vi "Error Query.vi"(8 "error in (no error)":errorcluster, 11 "VISA resource name":refnum<visa-resource-name>) -> (0 "error out":errorcluster, 1 "Error Message":string, 2 "Error Code":i32[](array[numeric]), 3 "VISA resource name out":refnum<visa-resource-name>)   [LabVIEW 2015, in "ZhiYuan ZDS Series for TCP.lvlib"]
doc: "Queries the instrument for any errors in the instrument's error queue. It will continue to read errors until all errors have been read from the instrument. Any errors will be returned in the <B>error out</B> control.\n\n<B>Note:</B>\nThis VI is called automatically by most driver VIs so it is not usually necessary to call this in an application."
uses:
  ZhiYuan ZDS Series for TCP.lvlib
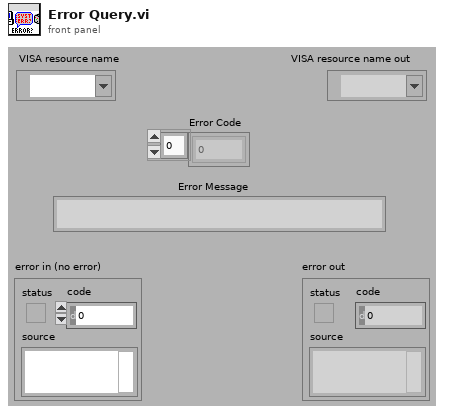
[diagram p1: front panel]
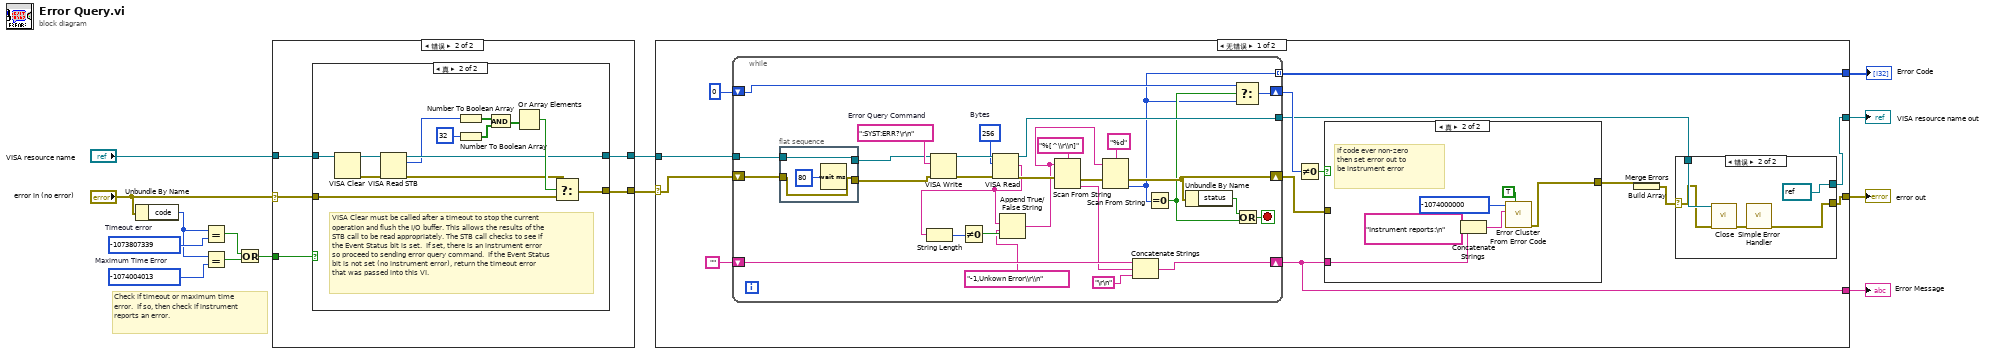
[diagram p0: block diagram]
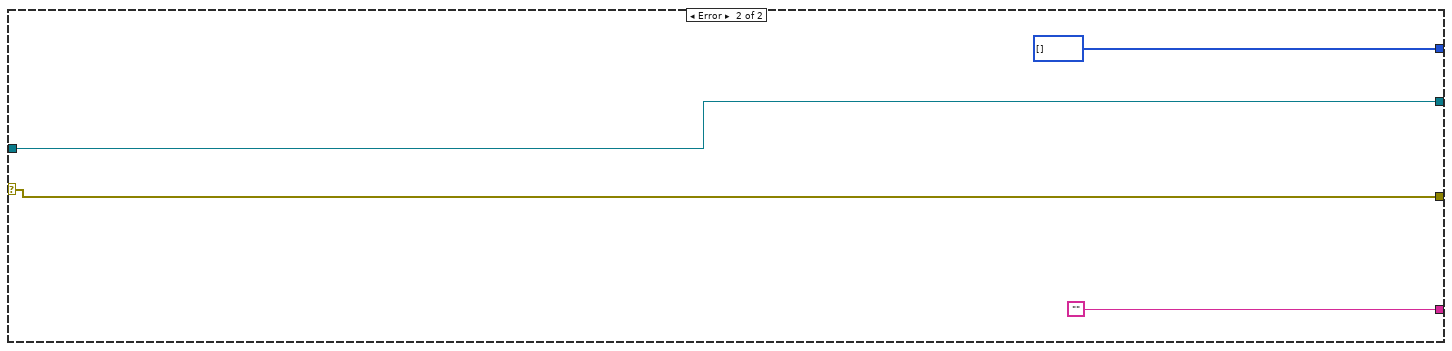
[diagram p6: hidden frame]
diagram:
  w5 = -1074004013  # Maximum Time Error
  w7 = -1073807339  # Timeout error
  # "Check if timeout or maximum time error.  If so, then check if instrument reports an error."
  n1 = Unbundle By Name("error in (no error)") -> ("code"=w6:i32)
  n2 = Equal?(x=w6, y=w7) -> (x = y?=w3:bool)
  n3 = Equal?(x=w6, y=w5) -> (x = y?=w4:bool)
  n4 = Or(x=w3, y=w4) -> (x .or. y?=w2:bool)
  n5 = case shown="错误" "error in (no error)" {
    selector: "error in (no error)" -> [w15 w19]
    tunnel: "VISA resource name" -> [w16 w21]
    tunnel: [w16 w20] -> w9
    tunnel: [w15 w18] -> w10
    tunnel: w2 -> [_ w17]
    frame No Error {
    }
    frame Error {
      n6 = case shown="真" w17 {
        tunnel: w21 -> [w23 w29]
        tunnel: [w23 w26] -> w20
        tunnel: w19 -> [w22 w32]
        tunnel: [w22 w31] -> w18
        frame False {
          # "Error code not a timeout, so best to pass on to user."
        }
        frame True {
          # "VISA Clear must be called after a timeout to stop the current operation and flush the I/O buffer. This allows the results of the  STB call to be read appropriately. The STB call checks to see if the Event Status bit is set.  If set, there is an instrument error so proceed to sending error query command.  If the Event Status bit is not set (no instrument error), return the timeout error that was passed into this VI."
          n7 = VISA Clear(VISA resource name=w29) -> (VISA resource name out=w28:refnum<visa-resource-name>, error out=w27:errorcluster)  [unwired: 1 in]
          n8 = VISA Read STB(8:w27, 11:w28) -> (0:w25:errorcluster, 2:w24:u16, 3:w26:refnum<visa-resource-name>)
          n9 = Number To Boolean Array(number=w24) -> (Boolean array=w33:bool[])
          n10 = Number To Boolean Array(number=32) -> (Boolean array=w35:bool[])
          n11 = And(x=w33, y=w35) -> (x .and. y?=w34:bool[])
          n12 = Or Array Elements(Boolean array=w34) -> (logical OR=w30:bool)
          n13 = Select(t=w25, s=w30, f=w32) -> (s? t:f=w31:errorcluster)
        }
      }
    }
  }
  n14 = case shown="无错误" w10 {
    selector: w10 -> [w42 w98]
    tunnel: [w37 w101] -> w14
    tunnel: w9 -> [w51 w101]
    tunnel: [w39 w98] -> w13
    tunnel: [w45 "" ("Empty String Constant")] -> w12
    tunnel: [w44 i32[] []] -> w11
    frame No Error {
      n15 = while {
        tunnel: [w94] -> w38
        tunnel: w51 -> [w69]
        shift-right: [w83] -> w45
        shift-left: "" ("Empty String Constant") -> [w86]
        shift-right: [w81] -> w46
        shift-left: 0 -> [w82]
        shift-right: [w80] -> w43
        shift-left: w42 -> [w68]
        tunnel: [w75] -> w44 mode=indexing
        stop <- w88 stop-if-true
        w92 = u32 256  # Bytes
        w90 = ":SYST:ERR?\r\n"  # Error Query Command
        n16 = flat-sequence {
          tunnel: w68 -> [w96]
          tunnel: [w95] -> w67
          tunnel: [w96] -> w66
          tunnel: w69 -> [w95]
          frame #0 {
            n17 = Wait (ms)(milliseconds to wait=u32 80 ("等待时间（毫秒）")) -> ()  [unwired: 1 out]
          }
        }
        n18 = VISA Write(VISA resource name=w67, write buffer=w90, error in (no error)=w66) -> (VISA resource name out=w93:refnum<visa-resource-name>, error out=w91:errorcluster)  [unwired: 1 out]
        n19 = VISA Read(VISA resource name=w93, byte count=w92, error in (no error)=w91) -> (VISA resource name out=w94:refnum<visa-resource-name>, read buffer=w72:string, error out=w79:errorcluster)  [unwired: 1 out]
        n20 = String Length(string=w72) -> (length=w74:i32)
        n21 = Not Equal To 0?(x=w74) -> (x != 0?=w73:bool)
        n22 = Append True/False String(1:w73, 2:"-1,Unkown Error\\r\\n", 3:w72) -> (0:w71:string)  [unwired: 1 in]
        n23 = Scan From String(format string="%[^\\r\\n]", input string=w71, error in=w79) -> (error out=w78:errorcluster, output 1=w84:string)  [unwired: 2 in, 2 out]
        n24 = Scan From String(format string="%d", input string=w71, error in=w78) -> (error out=w80:errorcluster, output 1=w75:i32)  [unwired: 2 in, 2 out]
        n25 = Concatenate Strings(w86, w84, "\r\n" ("End of Line Constant")) -> (w83:string)
        n26 = Equal To 0?(x=w75) -> (x = 0?=w76:bool)
        n27 = Unbundle By Name(w80) -> ("status"=w77:bool)
        n28 = Select(t=w82, s=w76, f=w75) -> (s? t:f=w81:i32)
        n29 = Or(x=w77, y=w76) -> (x .or. y?=w88:bool)
      }
      n30 = Not Equal To 0?(x=w46) -> (x != 0?=w48:bool)
      n31 = case shown="真" w48 {
        tunnel: w45 -> [_ w64]
        tunnel: [w59 w60] -> w47
        tunnel: w43 -> [w59 _]
        frame False {
        }
        frame True {
          # "If code ever non-zero\nthen set error out to\nbe instrument error"
          n32 = Concatenate Strings("Instrument reports:\n" ("Source"), w64) -> (w61:string)
          n33 = call <vilib>:"Error Cluster From Error Code.vi"("show call chain? (False)"=TRUE, "error message (\"\")"=w61, "error code (0)"=-1074000000 ("Code")) -> ("error out"=w60:errorcluster)  [unwired: 6 in]
        }
      }
      n34 = Build Array(w47) -> (w41:errorcluster[])
      n35 = Merge Errors(w41) -> (w40:errorcluster)
      n36 = case shown="错误" w40 {
        selector: w40 -> [w53 w55]
        tunnel: [w53 w54] -> w39
        tunnel: w38 -> [w52 w57]
        tunnel: [w52 refnum<visa-resource-name> refnum ("VISA resource name out")] -> w37
        frame No Error {
        }
        frame Error {
          n37 = call "Close.vi"("error in (no error)"=w55, "VISA resource name"=w57) -> ("error out"=w58:errorcluster)  [unwired: 9 in]
          n38 = call <vilib>:"Simple Error Handler.vi"("error in (no error)"=w58) -> ("error out"=w54:errorcluster)  [unwired: 4 in, 4 out]
        }
      }
    }
    frame Error {
    }
  }
  "VISA resource name out" <- w14
  "error out" <- w13
  "Error Message" <- w12
  "Error Code" <- w11
